vi "Settings.vi"(8 "error in (no error)":errorcluster, 11 "Crosshair Dispense in":refnum<class "Crosshair Dispense.lvclass">) -> (0 "error out":errorcluster, 3 "Crosshair Dispense out":refnum<class "Crosshair Dispense.lvclass">)   [LabVIEW 2019, in "Crosshair Dispense.lvclass"]
uses:
  Crosshair Dispense.lvclass
  Dispense.lvclass
panel:
  # "This Routine does not Accept Settings"
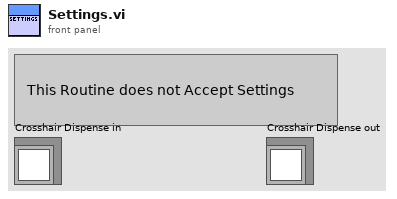
[diagram p1: front panel]
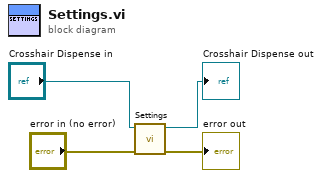
[diagram p0: block diagram]
diagram:
  n1 = call-parent "Settings.vi"("error in (no error)"="error in (no error)", "Routine in"="Crosshair Dispense in") -> ("error out"=→"error out":errorcluster, "Routine out"=→"Crosshair Dispense out":refnum<class "Crosshair Dispense.lvclass">)  [unwired: 8 in]
